vi "Sand Fall Till the Source Improved.vi"(3 "Possible Movements":cdb[](array[numeric]), 4 "Sand Source Coordinates":cdb, 5 "Rock Grid":set{cdb}(c389)) -> (0 "Bounds":T1, 1 "Sand Fall steps":T2(array[cluster]), 2 "Sand Grid":set{cdb}(c389))   [LabVIEW 2020, in "AoC 2022.lvlib"]
uses:
  AoC 2022.lvlib
  f83a1fb8-6652-4940-98ed-d4d1fe9cdb95.vi
  cd0c97e2-5f12-4d6f-9b1e-8c63b2a7a458.vi
  f83a1fb8-6652-4940-98ed-d4d1fe9cdb95.vi/7c7783df-fd5a-49d9-9b7a-63cc9fb0e4e5.vi
panel:
  out "size":i32
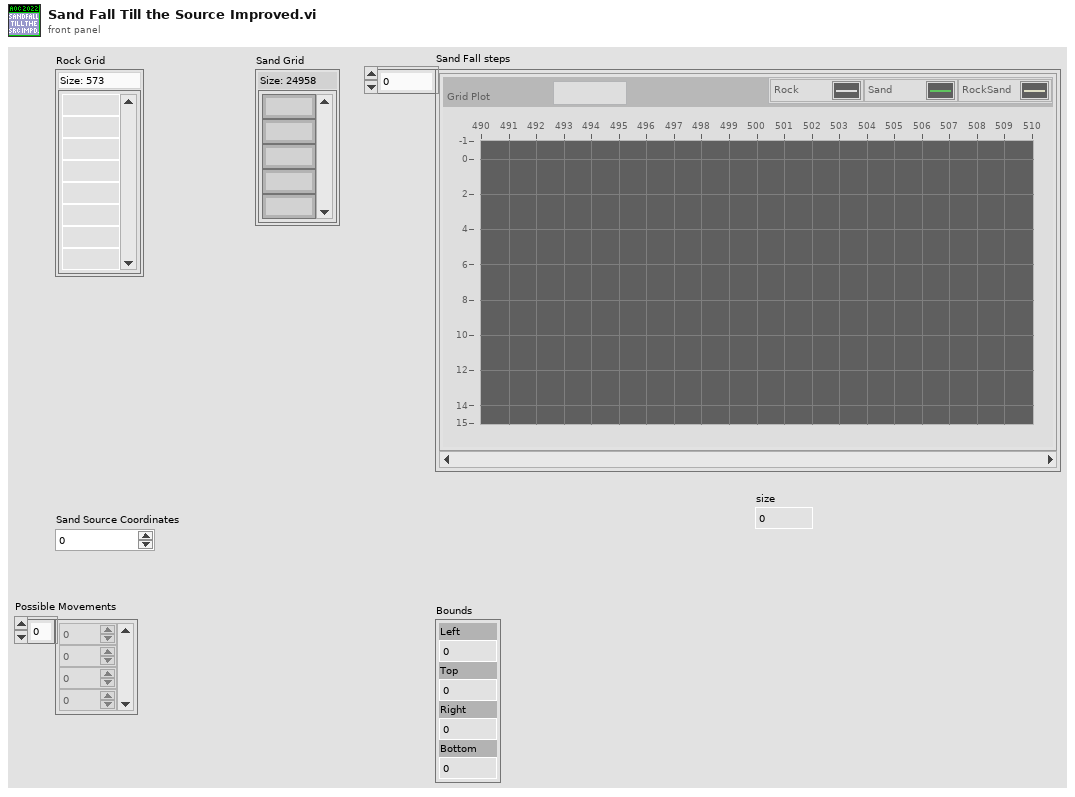
[diagram p1: front panel]
types:
  T1 = cluster{"Left":i16, "Top":i16, "Right":i16, "Bottom":i16}
  T2 = cluster{"Grid Plot":cluster{cluster{i32, i32}[]}[]}[]
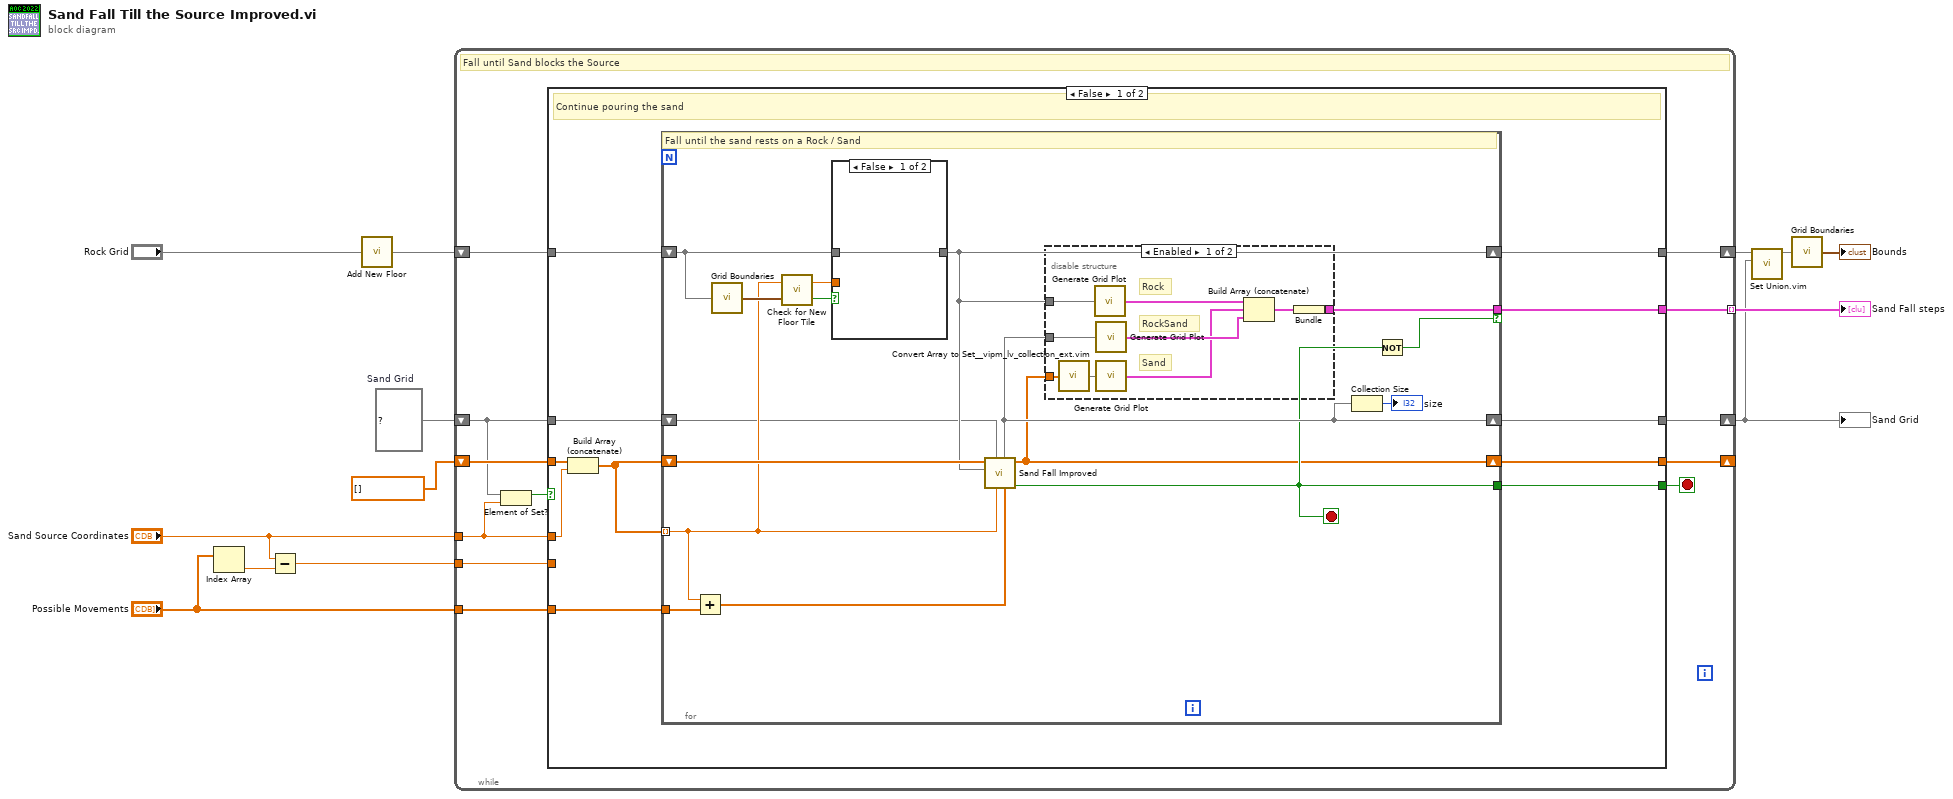
[diagram p0: block diagram]
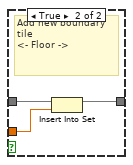
[diagram p3: hidden frame]
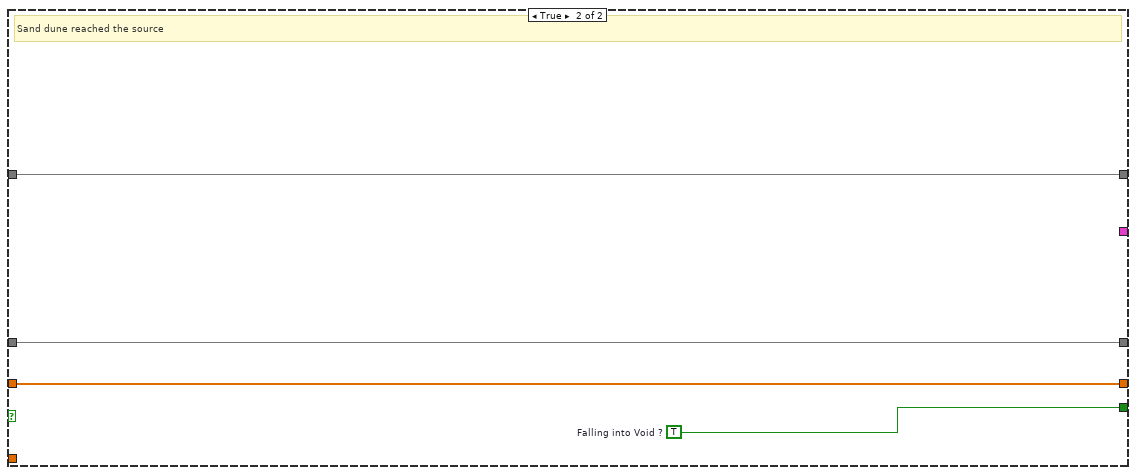
[diagram p4: hidden frame]
diagram:
  w8 = set{cdb} {}  # Sand Grid
  n1 = Index Array(array="Possible Movements") -> (element=w11:cdb)  [unwired: 1 in]
  n2 = Subtract(x="Sand Source Coordinates", y=w11) -> (x-y=w9:cdb)
  n3 = call "Add New Floor.vi"("Rock Grid in"="Rock Grid") -> ("Rock Grid out"=w7:set{cdb})
  n4 = while {
    shift-right: [w22] -> _
    shift-left: cdb[] [] ("Coordinates") -> [w19]
    tunnel: w9 -> [w15]
    tunnel: "Possible Movements" -> [w25]
    tunnel: [w23] -> w10 mode=indexing
    shift-right: [w20] -> w3
    shift-left: w7 -> [w21]
    tunnel: "Sand Source Coordinates" -> [w14]
    shift-right: [w17] -> w2
    shift-left: w8 -> [w16]
    stop <- w24 stop-if-true
    # "Fall until Sand blocks the Source"
    n5 = Element of Set?(10:w14, 11:w16) -> (3:w18:bool)
    n6 = case shown="False" w18 {
      tunnel: w25 -> [w36 _]
      tunnel: [w26 w68] -> w24
      tunnel: [w27 _] -> w23
      tunnel: [w35 w67] -> w22
      tunnel: w21 -> [w34 w69]
      tunnel: [w33 w69] -> w20
      tunnel: w19 -> [w30 w67]
      tunnel: w15 -> [_ _]
      tunnel: [w32 w66] -> w17
      tunnel: w16 -> [w31 w66]
      tunnel: w14 -> [w28 _]
      frame False {
        # "Continue pouring the sand"
        n7 = Build Array (concatenate)(w30, w28) -> (w29:cdb[])
        n8 = for {
          shift-right: [w38] -> w35
          shift-left: w29 -> [w45]
          tunnel: w36 -> [w52]
          tunnel: [w37] -> w27 if=w51
          shift-right: [w44] -> w33
          shift-left: w34 -> [w50]
          tunnel: w29 -> [w42] mode=indexing
          shift-right: [w40] -> w32
          shift-left: w31 -> [w41]
          tunnel: [w39] -> w26
          stop <- w39 stop-if-true
          # "Fall until the sand rests on a Rock / Sand"
          n9 = Add(x=w42, y=w52) -> (x+y=w43:cdb[])
          n10 = call "Grid Boundaries.vi"("Grid"=w50) -> ("Bounds"=w49:T1)
          n11 = call "Check for New Floor Tile.vi"("Bounds"=w49, "Current Location"=w42) -> ("Add floor tile ?"=w48:bool, "New Floor Tile"=w47:cdb)
          n12 = case shown="False" w48 {
            tunnel: w50 -> [w62 w65]
            tunnel: [w62 w64] -> w44
            tunnel: w47 -> [_ w63]
            frame False {
            }
            frame True {
              # "Add new boundary tile\n<- Floor ->"
              n13 = Insert Into Set(10:w63, 11:w65) -> (3:w64:set{cdb})  [unwired: 1 out]
            }
          }
          n14 = call "Sand Fall Improved.vi"("Next Possible Locations"=w43, "Current Sand Location"=w42, "RockSand Grid in"=w41, "Rock Grid"=w44, "Falling Sand List in"=w45) -> ("Falling into Void ?"=w39:bool, "Falling Sand List out"=w38:cdb[], "RockSand Grid out"=w40:set{cdb})  [unwired: 4 in]
          n15 = disable-structure shown="Enabled" {
            disable-tunnel: w44 -> [w61 _]
            disable-tunnel: w40 -> [w60 _]
            disable-tunnel: w38 -> [w59 _]
            disable-tunnel: [w57 _] -> w37
            frame Enabled {
              # "RockSand"
              # "Sand"
              # "Rock"
              n16 = call "Convert Array to Set__vipm_lv_collection_ext.vim"("array"=w59) -> ("set"=w58:set{cdb})  [unwired: 6 in]
              n17 = call "Generate Grid Plot.vi"("Grid"=w61) -> ("Grid Plot"=w56:cluster{cluster{i32, i32}[]}[])
              n18 = call "Generate Grid Plot.vi"("Grid"=w60) -> ("Grid Plot"=w54:cluster{cluster{i32, i32}[]}[])
              n19 = call "Generate Grid Plot.vi"("Grid"=w58) -> ("Grid Plot"=w53:cluster{cluster{i32, i32}[]}[])
              n20 = Build Array (concatenate)(w56, w53, w54) -> (w55:cluster{cluster{i32, i32}[]}[])
              n21 = Bundle(w55) -> (w57:cluster{cluster{cluster[]}[]})  [unwired: 1 in]
            }
            frame Disabled {
            }
          }
          n22 = Collection Size(1:w40) -> (0:→"size":i32)
          n23 = Not(x=w39) -> (.not. x?=w51:bool)
        }
      }
      frame True {
        w68 = TRUE  # Falling into Void ?
        # "Sand dune reached the source"
      }
    }
  }
  "Sand Grid" <- w2
  "Sand Fall steps" <- w10
  n24 = call "Set Union.vim"("set 2"=w2, "set 1"=w3) -> ("union"=w4:set{cdb})  [unwired: 9 in]
  n25 = call "Grid Boundaries.vi"("Grid"=w4) -> ("Bounds"=→"Bounds":T1)
